vi "class_data.vi"() -> ()   [LabVIEW 2010, in "FPGAWrapperDL090211Galvo.lvclass"]
uses:
  FPGAWrapperDL090211Galvo.lvclass
  FPGA_VI_ref.ctl
panel:
  in  "FPGA VI reference":T1
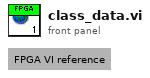
[diagram p1: front panel]
types:
  T1 = typedef "FPGAWrapperDL090211Galvo.lvclass/FPGA_VI_ref.ctl" = refnum<k20>
diagram:
